vi "CalcFeedForward.vi"(9 "Q":T1, 10 "B":T1, 11 "A":T1) -> (3 "Kff":T1)   [LabVIEW 2017]
uses:
  <vilib>/Analysis/Matrix/Datatypes/RealMatrix.ctl
  <vilib>/Analysis/_algsub.llb/Real PseudoInverse Matrix.vi
  <vilib>/Analysis/NI_AALPro.lvlib
  <vilib>/Analysis/Matrix/NI_Matrix.lvlib
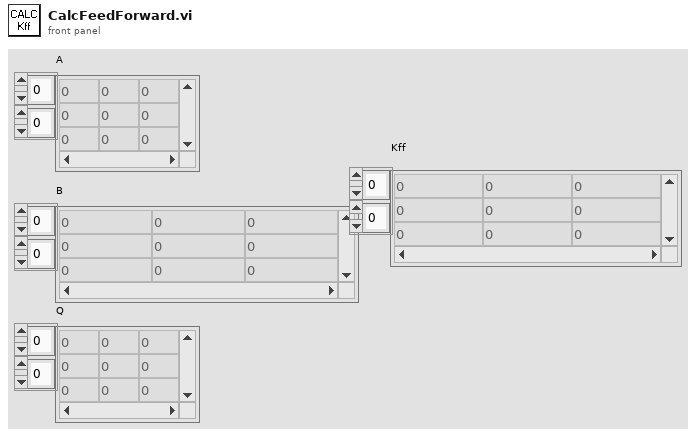
[diagram p1: front panel]
types:
  T1 = typedef "NI_Matrix.lvlib/RealMatrix.ctl" = dbl[][]
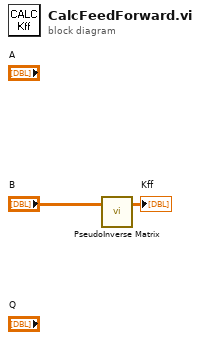
[diagram p0: block diagram]
diagram:
  n1 = call-poly <vilib>:"PseudoInverse Matrix.vi"("Input Matrix"="B") -> ("PseudoInverse Matrix"=→"Kff":T1)  [unwired: 1 in, 1 out]
